vi "Diagnostics.vi"(8 "error in (no error)":errorcluster, 10 "shutdown":refnum<user-event>, 11 "Modules":T5) -> (0 "Error 2":errorcluster)   [LabVIEW 2025]
uses:
  Libraries/USB IO/Classes/Hardware Selection.ctl
  Controls/Numeric Voltage.ctl
  Libraries/Power Supply/Classes/hardware-selection.ctl
  Controls/Numeric Current.ctl
  <vilib>/Handler Framework/CmdQueue/Enqueue Single.vi
  <vilib>/Handler Framework/Handler Framework.lvlib
  Libraries/USB IO/USB IO.lvlib
  Libraries/Power Supply/Power Supply.lvlib
panel:
  out "Amps":T1 format="%5.3f A"
  out "Volts":T2 format="%5.3f V"
  in  "Set Output":bool
  in  "Set Current":bool
  in  "Output Current":dbl=0.05
  in  "Set Voltage":bool
  in  "Output Voltage":dbl=10.0
  in  "VISA Instrument":refnum<visa-resource-name>="N/A"
  in  "PS Reconnect":bool
  in  "Power Supply":T3=enum."PSP-603"
  out "Voltage Chart":dbl(graph)
  in  "Digital Value":bool
  in  "Write":bool
  out "Voltage":T2 format="%5.3f V"
  in  "Read":bool
  in  "Lines":u16(ring)
  in  "I/O Reconnect":bool
  in  "Serial Port":refnum<visa-resource-name>="N/A"
  in  "I/O Device":T4=enum."USB-6000"
  out "Module Names":string[](array[string])
  out "Error":errorcluster
  # "Diagnostics"
  # "Modules"
  # "USB I/O"
  # "POWER SUPPLY"
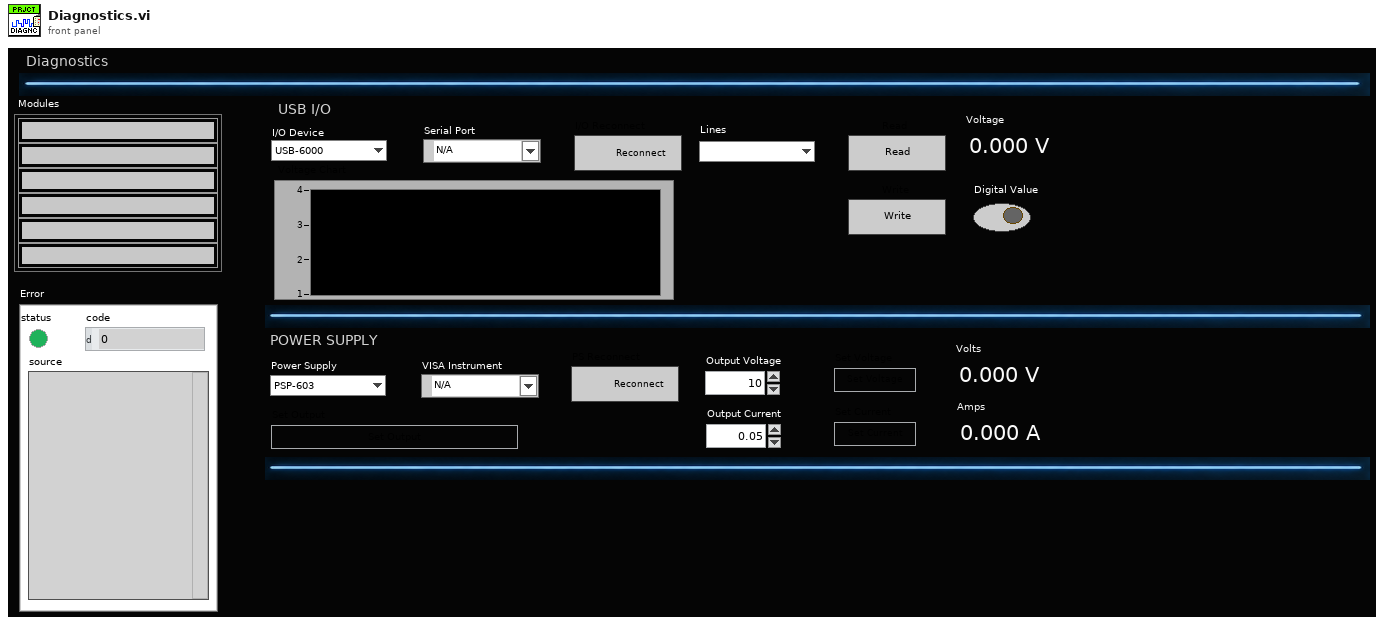
[diagram p1: front panel]
types:
  T1 = typedef "Numeric Current.ctl" = dbl
  T2 = typedef "Numeric Voltage.ctl" = dbl
  T3 = typedef "hardware-selection.ctl" = enum16{"Parent", "Simulation", "PSP-603"}
  T4 = typedef "Hardware Selection.ctl" = enum16{"Simulation", "USB-6000", "USB-6001", "Arduino Uno"}
  T5 = cluster{"Module IDs":i32[], "Module Names":string[]}
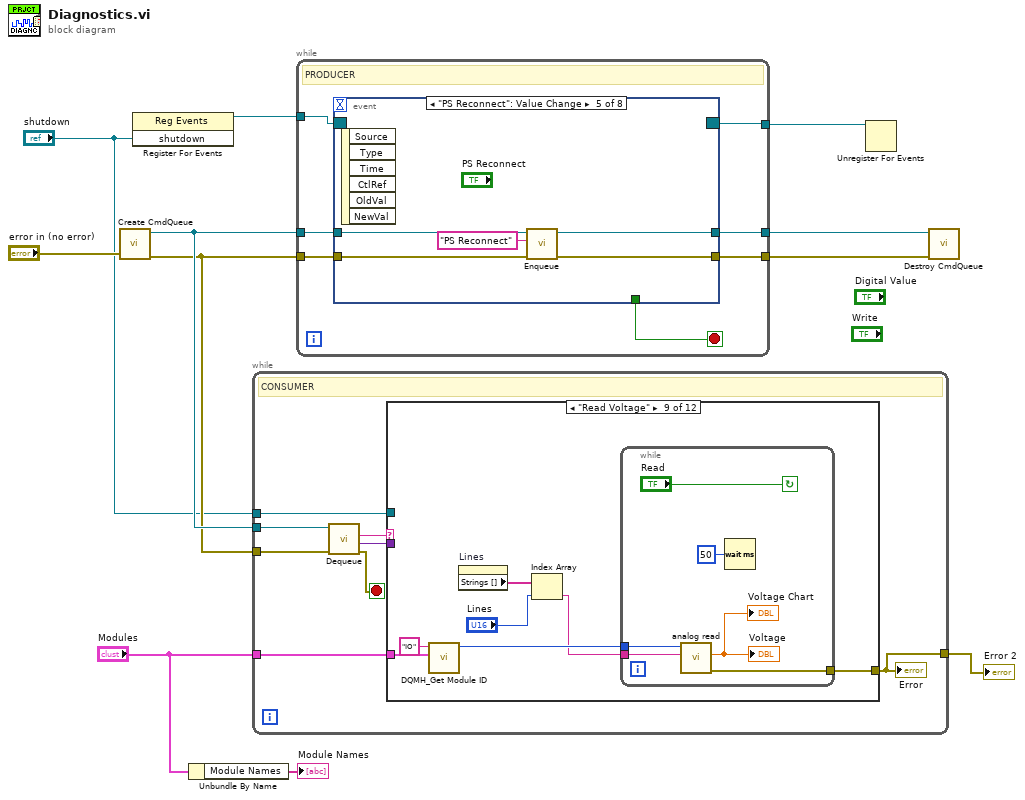
[diagram p0: block diagram]
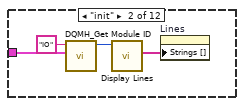
[diagram p3: hidden frame]
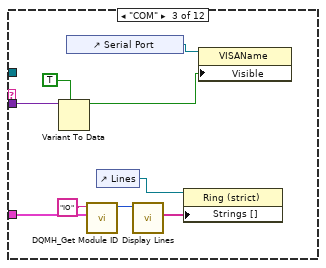
[diagram p4: hidden frame]
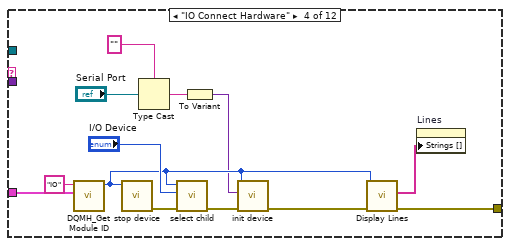
[diagram p5: hidden frame]
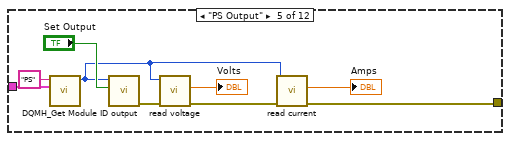
[diagram p6: hidden frame]
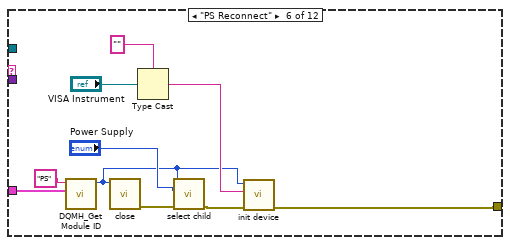
[diagram p7: hidden frame]
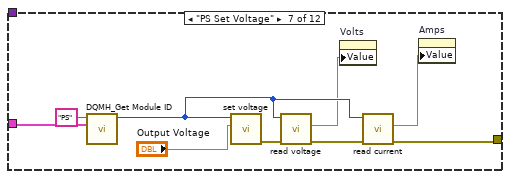
[diagram p8: hidden frame]
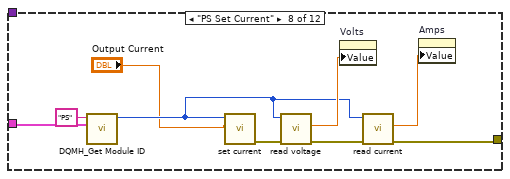
[diagram p9: hidden frame]
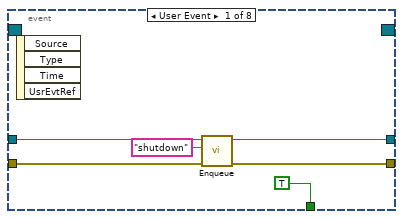
[diagram p13: hidden frame]
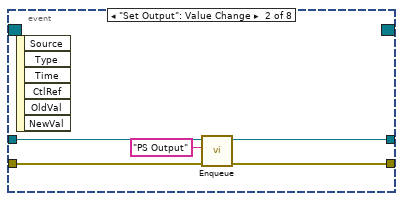
[diagram p14: hidden frame]
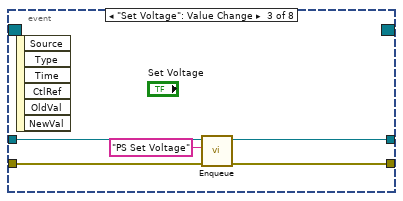
[diagram p15: hidden frame]
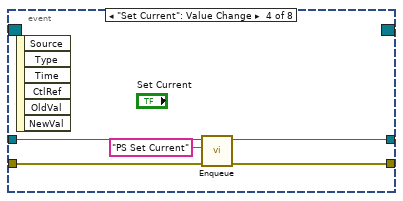
[diagram p16: hidden frame]
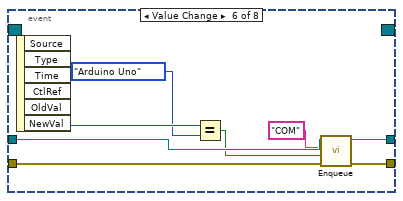
[diagram p17: hidden frame]
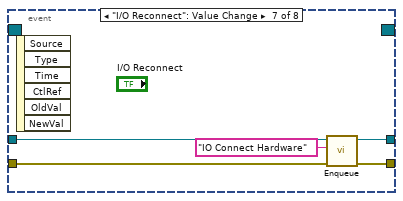
[diagram p18: hidden frame]
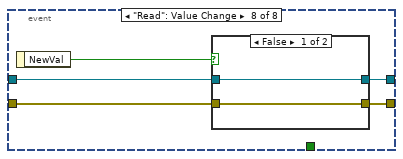
[diagram p19: hidden frame]
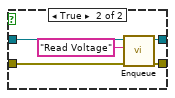
[diagram p20: hidden frame]
diagram:
  n1 = call <vilib>:"Create CmdQueue.vi"("error in (no error)"="error in (no error)") -> ("error out"=w8:errorcluster, "CmdQueue out"=w9:refnum<queue>)  [unwired: 9 in]
  n2 = register-events("shutdown") -> (reference out=w7:refnum<event-registration>)  [unwired: 2 in, 1 out]
  n3 = Unbundle By Name("Modules") -> ("Module Names"=→"Module Names":string[])
  n4 = while {
    tunnel: w9 -> [w19]
    tunnel: w8 -> [w15]
    tunnel: "shutdown" -> [w14]
    tunnel: "Modules" -> [w13]
    tunnel: [w12] -> w1
    stop <- w16 stop-if-true
    # "CONSUMER"
    n5 = call <vilib>:"Dequeue.vi"("error in (no error)"=w15, "CmdQueue in"=w19) -> ("error out"=w16:errorcluster, "value"=w17:variant, "cmd"=w18:string)  [unwired: 5 in, 2 out]
    n6 = case shown="\"Read Voltage\"" w18 {
      tunnel: w17 -> [_ _ w31 _ _ _ _ _ _ _ _ _]
      tunnel: w14 -> [_ _ _ _ _ _ _ _ _ _ _ _]
      tunnel: w13 -> [_ w23 w25 w45 w54 w63 w72 w81 w89 _ _ _]
      tunnel: [_ _ _ w33 w47 w55 w65 w77 w83 _ _ _] -> w12
      frame "False", Default {
      }
      frame "init" {
        n7 = call "DQMH_Get Module ID.vi"("Modules"=w23, "Module Name"="IO") -> ("Module ID out"=w21:i32)  [unwired: 9 in]
        n8 = call "Display Lines.vi"("Module ID"=w21) -> ("Lines"=w20:string[])  [unwired: 7 in, 3 out]
        n9 = property on="Lines" class="Ring (strict)"("Strings []"=w20) -> ()  [unwired: 2 in, 2 out]
      }
      frame "COM" {
        n10 = Variant To Data(type=TRUE, Variant=w31) -> (data=w29:bool)  [unwired: 1 in, 1 out]
        n11 = control-ref of="Serial Port"() -> (w32:refnum<vi>)
        n12 = call "DQMH_Get Module ID.vi"("Modules"=w25, "Module Name"="IO") -> ("Module ID out"=w27:i32)  [unwired: 9 in]
        n13 = control-ref of="Lines"() -> (w24:refnum<vi>)
        n14 = call "Display Lines.vi"("Module ID"=w27) -> ("Lines"=w26:string[])  [unwired: 7 in, 3 out]
        n15 = property on="Property Node" class="Ring (strict)"(reference=w24, "Strings []"=w26) -> ()  [unwired: 1 in, 2 out]
        n16 = property class="VISAName"(reference=w32, "Visible"=w29) -> ()  [unwired: 1 in, 2 out]
      }
      frame "IO Connect Hardware" {
        n17 = call "DQMH_Get Module ID.vi"("Modules"=w45, "Module Name"="IO") -> ("Module ID out"=w42:i32)  [unwired: 9 in]
        n18 = call "stop device.vi"("Module ID"=w42) -> ("error out"=w36:errorcluster)  [unwired: 9 in, 1 out]
        n19 = Type Cast(type="", x="Serial Port") -> (*(type *) &x=w38:string)
        n20 = call "select child.vi"("error in"=w36, "Hardware"="I/O Device", "Module ID"=w42) -> ("error out"=w34:errorcluster)  [unwired: 7 in, 1 out]
        n21 = To Variant(anything=w38) -> (Variant=w37:variant)
        n22 = call "init device.vi"("error in"=w34, "Variant"=w37, "Module ID"=w42) -> ("error out"=w35:errorcluster)  [unwired: 7 in, 1 out]
        n23 = call "Display Lines.vi"("error in"=w35, "Module ID"=w42) -> ("error out"=w33:errorcluster, "Lines"=w41:string[])  [unwired: 6 in, 2 out]
        n24 = property on="Lines" class="Ring (strict)"("Strings []"=w41) -> ()  [unwired: 2 in, 2 out]
      }
      frame "PS Output" {
        n25 = call "DQMH_Get Module ID.vi"("Modules"=w54, "Module Name"="PS") -> ("Module ID out"=w48:i32)  [unwired: 9 in]
        n26 = call "output.vi"("Output On/Off"="Set Output", "Module ID"=w48) -> ("error out"=w51:errorcluster)  [unwired: 8 in, 1 out]
        n27 = call "read voltage.vi"("error in"=w51, "Module ID"=w48) -> ("error out"=w49:errorcluster, "Volts"=→"Volts":T2)  [unwired: 7 in, 1 out]
        n28 = call "read current.vi"("error in"=w49, "Module ID"=w48) -> ("error out"=w47:errorcluster, "Amps"=→"Amps":T1)  [unwired: 7 in, 1 out]
      }
      frame "PS Reconnect" {
        n29 = call "DQMH_Get Module ID.vi"("Modules"=w63, "Module Name"="PS") -> ("Module ID out"=w56:i32)  [unwired: 9 in]
        n30 = call "close.vi"("Module ID"=w56) -> ("error out"=w62:errorcluster)  [unwired: 9 in, 1 out]
        n31 = Type Cast(type="", x="VISA Instrument") -> (*(type *) &x=w58:string)
        n32 = call "select child.vi"("error in"=w62, "Enum"="Power Supply", "Module ID"=w56) -> ("error out"=w57:errorcluster)  [unwired: 7 in, 1 out]
        n33 = call "init device.vi"("error in"=w57, "Variant"=w58, "Module ID"=w56) -> ("error out"=w55:errorcluster)  [unwired: 7 in, 1 out]
      }
      frame "PS Set Voltage" {
        n34 = call "DQMH_Get Module ID.vi"("Modules"=w72, "Module Name"="PS") -> ("Module ID out"=w68:i32)  [unwired: 9 in]
        n35 = call "set voltage.vi"("Output Voltage"="Output Voltage", "Module ID"=w68) -> ("error out"=w70:errorcluster)  [unwired: 8 in, 1 out]
        n36 = call "read voltage.vi"("error in"=w70, "Module ID"=w68) -> ("error out"=w69:errorcluster, "Volts"=w67:T2)  [unwired: 7 in, 1 out]
        n37 = property on="Volts" class="DigNum (strict)"("Value"=w67) -> ()  [unwired: 2 in, 2 out]
        n38 = call "read current.vi"("error in"=w69, "Module ID"=w68) -> ("error out"=w65:errorcluster, "Amps"=w66:T1)  [unwired: 7 in, 1 out]
        n39 = property on="Amps" class="DigNum (strict)"("Value"=w66) -> ()  [unwired: 2 in, 2 out]
      }
      frame "PS Set Current" {
        n40 = call "DQMH_Get Module ID.vi"("Modules"=w81, "Module Name"="PS") -> ("Module ID out"=w75:i32)  [unwired: 9 in]
        n41 = call "set current.vi"("Output Current"="Output Current", "Module ID"=w75) -> ("error out"=w76:errorcluster)  [unwired: 8 in, 1 out]
        n42 = call "read voltage.vi"("error in"=w76, "Module ID"=w75) -> ("error out"=w80:errorcluster, "Volts"=w79:T2)  [unwired: 7 in, 1 out]
        n43 = property on="Volts" class="DigNum (strict)"("Value"=w79) -> ()  [unwired: 2 in, 2 out]
        n44 = call "read current.vi"("error in"=w80, "Module ID"=w75) -> ("error out"=w77:errorcluster, "Amps"=w78:T1)  [unwired: 7 in, 1 out]
        n45 = property on="Amps" class="DigNum (strict)"("Value"=w78) -> ()  [unwired: 2 in, 2 out]
      }
      frame "Read Voltage" {
        n46 = call "DQMH_Get Module ID.vi"("Modules"=w89, "Module Name"="IO") -> ("Module ID out"=w87:i32)  [unwired: 9 in]
        n47 = property on="Lines" class="Ring (strict)"() -> ("Strings []"=w86:string[])  [unwired: 2 in, 2 out]
        n48 = Index Array(array=w86, index="Lines") -> (element=w84:string)
        n49 = while {
          tunnel: w87 -> [w95]
          tunnel: w84 -> [w94]
          tunnel: [w93] -> w83
          stop <- "Read" continue-if-true
          n50 = call "analog read.vi"("Line"=w94, "Module ID"=w95) -> ("error out"=w93:errorcluster, "Voltage"=→"Voltage" →"Voltage Chart":T2)  [unwired: 7 in, 1 out]
          n51 = Wait (ms)(milliseconds to wait=u32 50) -> ()  [unwired: 1 out]
        }
      }
      frame "shutdown" {
      }
      frame "append" {
      }
      frame "save & clear" {
      }
    }
    "Error" <- w12
  }
  "Error 2" <- w1
  n52 = while {
    tunnel: w9 -> [w102]
    tunnel: [w101] -> w11
    tunnel: w8 -> [w100]
    tunnel: [w99] -> w10
    tunnel: w7 -> [w97]
    tunnel: [w96] -> w6
    stop <- w98 stop-if-true
    # "PRODUCER"
    n53 = event shown="[4] \"PS Reconnect\": Value Change" {
      selector: w97 -> [_ _ _ _ _ _ _ _]
      dyn-events: [_ _ _ _ _ _ _ _] -> w96
      timeout: _ -> [_ _ _ _ _ _ _ _]
      tunnel: w102 -> [w108 w113 w118 w123 w128 w132 w139 w144]
      tunnel: [w107 w112 w117 w122 w127 w133 w140 w145] -> w101
      tunnel: w100 -> [w106 w111 w116 w121 w126 w131 w138 w143]
      tunnel: [w105 w110 w115 w120 w125 w134 w141 w146] -> w99
      tunnel: [TRUE ("Discard?") _ _ _ _ _ _ _] -> w98
      event User Event {
        n54 = event-data() -> ()  [unwired: 1 in, 4 out]
        n55 = call-poly <vilib>:"Enqueue.vi"("error in (no error)"=w106, "Command"="shutdown", "CmdQueue in"=w108) -> ("error out"=w105:errorcluster, "CmdQueue out"=w107:refnum<queue>)  [unwired: 7 in]
      }
      event "Set Output": Value Change {
        n56 = event-data() -> ()  [unwired: 1 in, 6 out]
        n57 = call-poly <vilib>:"Enqueue.vi"("error in (no error)"=w111, "Command"="PS Output", "CmdQueue in"=w113) -> ("error out"=w110:errorcluster, "CmdQueue out"=w112:refnum<queue>)  [unwired: 7 in]
      }
      event "Set Voltage": Value Change {
        n58 = event-data() -> ()  [unwired: 1 in, 6 out]
        n59 = call-poly <vilib>:"Enqueue.vi"("error in (no error)"=w116, "Command"="PS Set Voltage", "CmdQueue in"=w118) -> ("error out"=w115:errorcluster, "CmdQueue out"=w117:refnum<queue>)  [unwired: 7 in]
      }
      event "Set Current": Value Change {
        n60 = event-data() -> ()  [unwired: 1 in, 6 out]
        n61 = call-poly <vilib>:"Enqueue.vi"("error in (no error)"=w121, "Command"="PS Set Current", "CmdQueue in"=w123) -> ("error out"=w120:errorcluster, "CmdQueue out"=w122:refnum<queue>)  [unwired: 7 in]
      }
      event "PS Reconnect": Value Change {
        n62 = event-data() -> ()  [unwired: 1 in, 6 out]
        n63 = call-poly <vilib>:"Enqueue.vi"("error in (no error)"=w126, "Command"="PS Reconnect", "CmdQueue in"=w128) -> ("error out"=w125:errorcluster, "CmdQueue out"=w127:refnum<queue>)  [unwired: 7 in]
      }
      event Value Change {
        n64 = event-data() -> ("NewVal"=w136:T4)  [unwired: 1 in, 5 out]
        n65 = Equal?(x=w136, y=Hardware_Selection."Arduino Uno" ("NewVal")) -> (x = y?=w129:bool)
        n66 = call-poly <vilib>:"Enqueue.vi"("error in (no error)"=w131, "Value"=w129, "Command"="COM", "CmdQueue in"=w132) -> ("error out"=w134:errorcluster, "CmdQueue out"=w133:refnum<queue>)  [unwired: 6 in]
      }
      event "I/O Reconnect": Value Change {
        n67 = event-data() -> ()  [unwired: 1 in, 6 out]
        n68 = call-poly <vilib>:"Enqueue.vi"("error in (no error)"=w138, "Command"="IO Connect Hardware", "CmdQueue in"=w139) -> ("error out"=w141:errorcluster, "CmdQueue out"=w140:refnum<queue>)  [unwired: 7 in]
      }
      event "Read": Value Change {
        n69 = event-data() -> ("NewVal"=w142:bool)  [unwired: 1 in]
        n70 = case shown="False" w142 {
          tunnel: [w147 w153] -> w146
          tunnel: [w148 w152] -> w145
          tunnel: w144 -> [w148 w151]
          tunnel: w143 -> [w147 w150]
          frame False {
          }
          frame True {
            n71 = call-poly <vilib>:"Enqueue.vi"("error in (no error)"=w150, "Command"="Read Voltage", "CmdQueue in"=w151) -> ("error out"=w153:errorcluster, "CmdQueue out"=w152:refnum<queue>)  [unwired: 7 in]
          }
        }
      }
    }
  }
  n72 = Unregister For Events(event registration refnum=w6) -> ()  [unwired: 1 in, 1 out]
  n73 = call <vilib>:"Destroy CmdQueue.vi"("error in (no error)"=w10, "CmdQueue in"=w11) -> ()  [unwired: 9 in, 1 out]
